vi "Sort 1D Array PtByPt.vi"(2 "initialize":bool, 3 "sample length":i32=100, 5 "input data point":dbl format="%0.2f") -> (0 "error":i32, 1 "sorted array":dbl[](array[numeric]))   [LabVIEW 2020, in "NI_PtbyPt.lvlib"]
doc: "Sorts the set of input data points specified by <B>sample length</B> in ascending order."
uses:
  NI_PtbyPt.lvlib
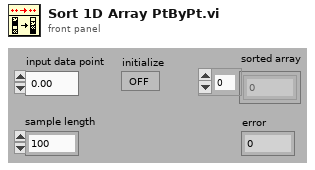
[diagram p1: front panel]
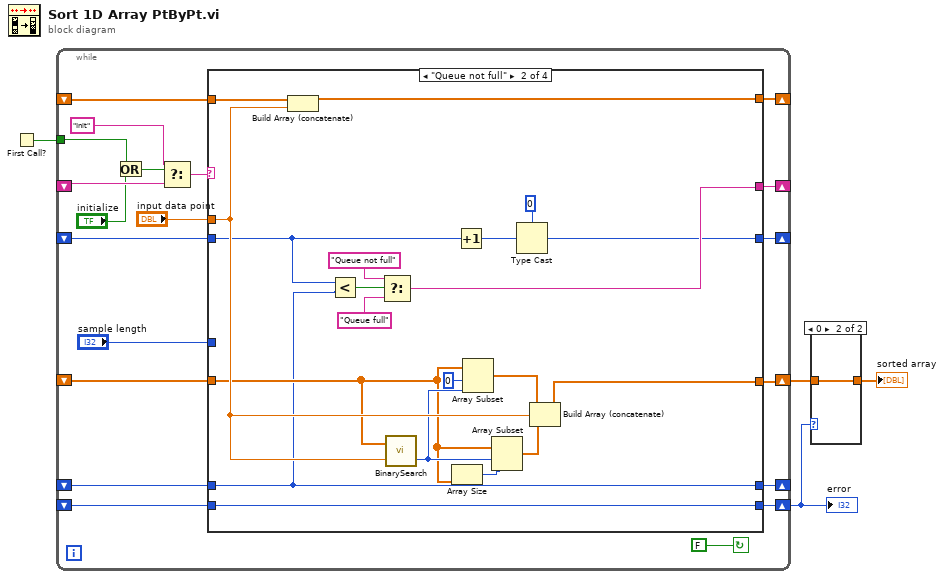
[diagram p0: block diagram]
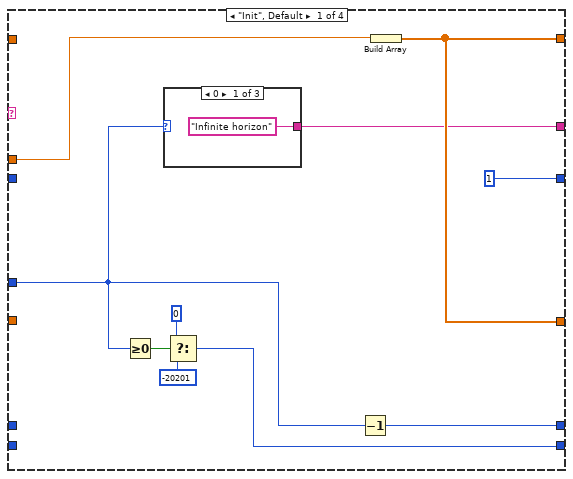
[diagram p3: hidden frame]
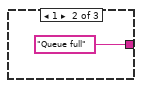
[diagram p4: hidden frame]
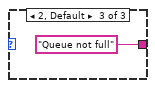
[diagram p5: hidden frame]
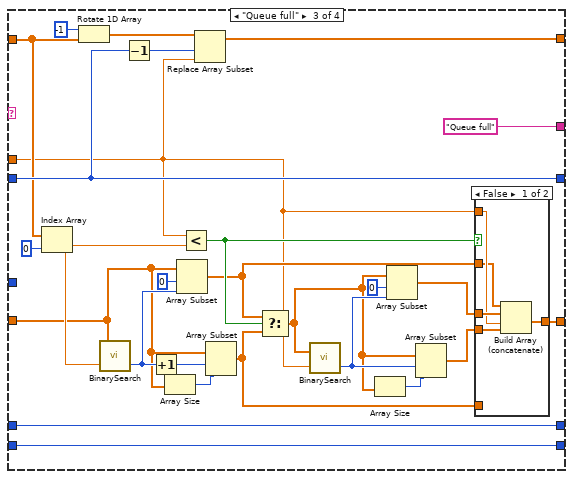
[diagram p6: hidden frame]
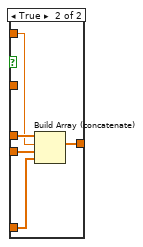
[diagram p7: hidden frame]
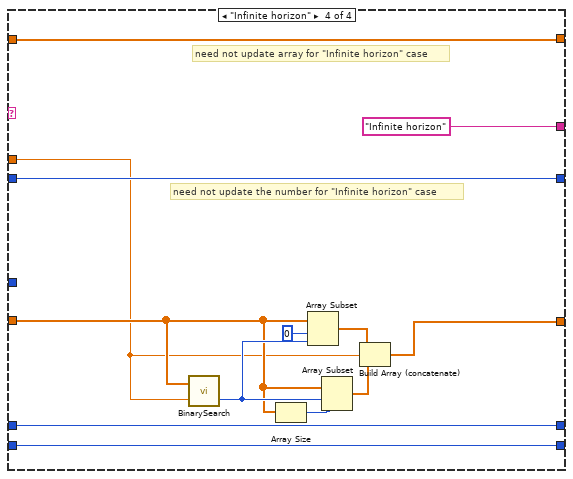
[diagram p8: hidden frame]
diagram:
  n1 = First Call?() -> (First Call?: T/F=w4:bool)
  n2 = while {
    shift-left: _ -> [w7]
    shift-right: [w8] -> _
    tunnel: w4 -> [w10]
    shift-left: _ -> [w15]
    shift-right: [w16] -> _
    shift-left: _ -> [w18]
    shift-right: [w19] -> _
    shift-left: _ -> [w23]
    shift-right: [w20] -> _
    shift-left: _ -> [w14]
    shift-right: [w13] -> w2
    shift-right: [w6] -> w3
    shift-left: _ -> [w5]
    stop <- FALSE continue-if-true
    n3 = Or(x=w10, y="initialize") -> (x .or. y?=w11:bool)
    n4 = Select(t="Init", s=w11, f=w23) -> (s? t:f=w22:string)
    n5 = case shown="\"Queue not full\"" w22 {
      tunnel: "sample length" -> [w25 _ _ _]
      tunnel: [w26 w54 "Queue full" "Infinite horizon"] -> w20
      tunnel: [1 w52 w81 w106] -> w19
      tunnel: w18 -> [_ w40 w81 w106]
      tunnel: "input data point" -> [w33 w48 w60 w97]
      tunnel: [w32 w49 w79 w105] -> w16
      tunnel: w15 -> [_ w50 w74 w105]
      tunnel: w14 -> [_ w42 w71 w99]
      tunnel: [w32 w41 w65 w98] -> w13
      tunnel: [w28 w39 w59 w96] -> w8
      tunnel: w7 -> [_ w39 w59 w96]
      tunnel: [w27 w38 w58 w95] -> w6
      tunnel: w5 -> [_ w38 w58 w95]
      frame "Init", Default {
        n6 = Greater Or Equal To 0?(x=w25) -> (x >= 0?=w29:bool)
        n7 = case shown="0" w25 {
          tunnel: ["Infinite horizon" "Queue full" "Queue not full"] -> w26
          frame 0 {
          }
          frame 1 {
          }
          frame 2, Default {
          }
        }
        n8 = Select(t=0, s=w29, f=-20201) -> (s? t:f=w27:i32)
        n9 = Decrement(x=w25) -> (x-1=w28:i32)
        n10 = Build Array(w33) -> (w32:dbl[])
      }
      frame "Queue not full" {
        n11 = Build Array (concatenate)(w50, w48) -> (w49:dbl[])
        n12 = Less?(x=w40, y=w39) -> (x < y?=w57:bool)
        n13 = Select(t="Queue not full", s=w57, f="Queue full") -> (s? t:f=w54:string)
        n14 = call "BinarySearch.vi"("value searching for"=w48, "Sorted Array"=w42) -> ("index"=w45:i32)  [unwired: 1 out]
        n15 = Array Size(array=w42) -> (size(s)=w44:i32)
        n16 = Increment(x=w40) -> (x+1=w53:i32)
        n17 = Array Subset(array=w42, index=0 ("Array Index"), length=w45) -> (w47:dbl[])
        n18 = Array Subset(array=w42, index=w45, length=w44) -> (w46:dbl[])
        n19 = Type Cast(type=0, x=w53) -> (*(type *) &x=w52:i32)
        n20 = Build Array (concatenate)(w47, w48, w46) -> (w41:dbl[])
      }
      frame "Queue full" {
        n21 = Index Array(array=w74, index=0 ("Index")) -> (element=w72:dbl)
        n22 = Rotate 1D Array(1:w74, 2:i16 -1 ("n")) -> (0:w82:dbl[])
        n23 = call "BinarySearch.vi"("value searching for"=w72, "Sorted Array"=w71) -> ("index"=w76:i32)  [unwired: 1 out]
        n24 = Decrement(x=w81) -> (x-1=w80:i32)
        n25 = Increment(x=w76) -> (x+1=w77:i32)
        n26 = Array Size(array=w71) -> (size(s)=w78:i32)
        n27 = Array Subset(array=w71, index=0 ("Array Index"), length=w76) -> (w62:dbl[])
        n28 = Less?(x=w60, y=w72) -> (x < y?=w63:bool)
        n29 = Replace Array Subset(array=w82, new element=w60, index=w80) -> (w79:dbl[])
        n30 = Array Subset(array=w71, index=w77, length=w78) -> (w61:dbl[])
        n31 = Select(t=w62, s=w63, f=w61) -> (s? t:f=w64:dbl[])
        n32 = call "BinarySearch.vi"("value searching for"=w60, "Sorted Array"=w64) -> ("index"=w68:i32)  [unwired: 1 out]
        n33 = Array Size(array=w64) -> (size(s)=w67:i32)
        n34 = Array Subset(array=w64, index=0 ("Array Index"), length=w68) -> (w70:dbl[])
        n35 = Array Subset(array=w64, index=w68, length=w67) -> (w69:dbl[])
        n36 = case shown="False" w63 {
          tunnel: w70 -> [w89 w93]
          tunnel: w69 -> [w88 w92]
          tunnel: [w86 w94] -> w65
          tunnel: w62 -> [w85 _]
          tunnel: w61 -> [_ w90]
          tunnel: w60 -> [w87 w91]
          frame False {
            n37 = Build Array (concatenate)(w85, w89, w87, w88) -> (w86:dbl[])
          }
          frame True {
            n38 = Build Array (concatenate)(w93, w91, w92, w90) -> (w94:dbl[])
          }
        }
      }
      frame "Infinite horizon" {
        # "need not update the number for \"Infinite horizon\" case"
        # "need not update array for \"Infinite horizon\" case"
        n39 = call "BinarySearch.vi"("value searching for"=w97, "Sorted Array"=w99) -> ("index"=w102:i32)  [unwired: 1 out]
        n40 = Array Size(array=w99) -> (size(s)=w101:i32)
        n41 = Array Subset(array=w99, index=0 ("Array Index"), length=w102) -> (w104:dbl[])
        n42 = Array Subset(array=w99, index=w102, length=w101) -> (w103:dbl[])
        n43 = Build Array (concatenate)(w104, w97, w103) -> (w98:dbl[])
      }
    }
  }
  "error" <- w3
  n44 = case shown="0" w3 {
    tunnel: w2 -> [_ w108]
    tunnel: [_ w108] -> w1
    frame -1, Default {
    }
    frame 0 {
    }
  }
  "sorted array" <- w1
